vi "FTW-NUM-Increment.vi"(0 "Initial Value":i32 format="%08x", 1 "Increment?":bool) -> (2 "Final Value":i32 format="%08x")   [LabVIEW 2013]
panel:
  # "Inputs"
  # "Outputs"
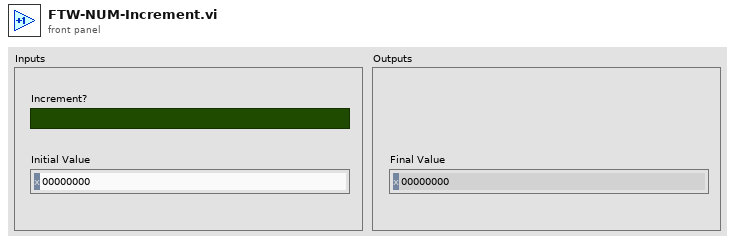
[diagram p1: front panel]
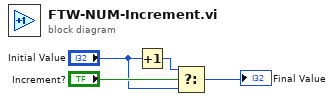
[diagram p0: block diagram]
diagram:
  n1 = Increment(x="Initial Value") -> (x+1=w2:i32)
  n2 = Select(t=w2, s="Increment?", f="Initial Value") -> (s? t:f=→"Final Value":i32)
